vi "AIT 664 - Read End System XML.vi"(0 "Refnum in":refnum<k20>, 11 "error in (no error)":errorcluster) -> (4 "664 End System":T1, 15 "error out":errorcluster)   [LabVIEW 2013, in "AIT 664 Custom Device.lvlib"]
doc: "Read all of the nodes of the end system from xml configuration"
uses:
  AIT 664 Custom Device.lvlib
  Controls/664 - XML End System Description.ctl
  Controls/664 - XML Output VL.ctl
  Controls/664 - XML Tx Message Port.ctl
  Controls/664 - Sampling Type.ctl
  Controls/664 -Param.ctl
  Controls/664 - XML Input VL.ctl
  Controls/664 - XML Rx Message Port.ctl
  <vilib>/xml/Close Reference(NNMap).vi
  <vilib>/xml/Close Reference(Node).vi
  <resource>/objmgr/DOMUserDefRef.rc
  <vilib>/xml/NI_XML.lvlib
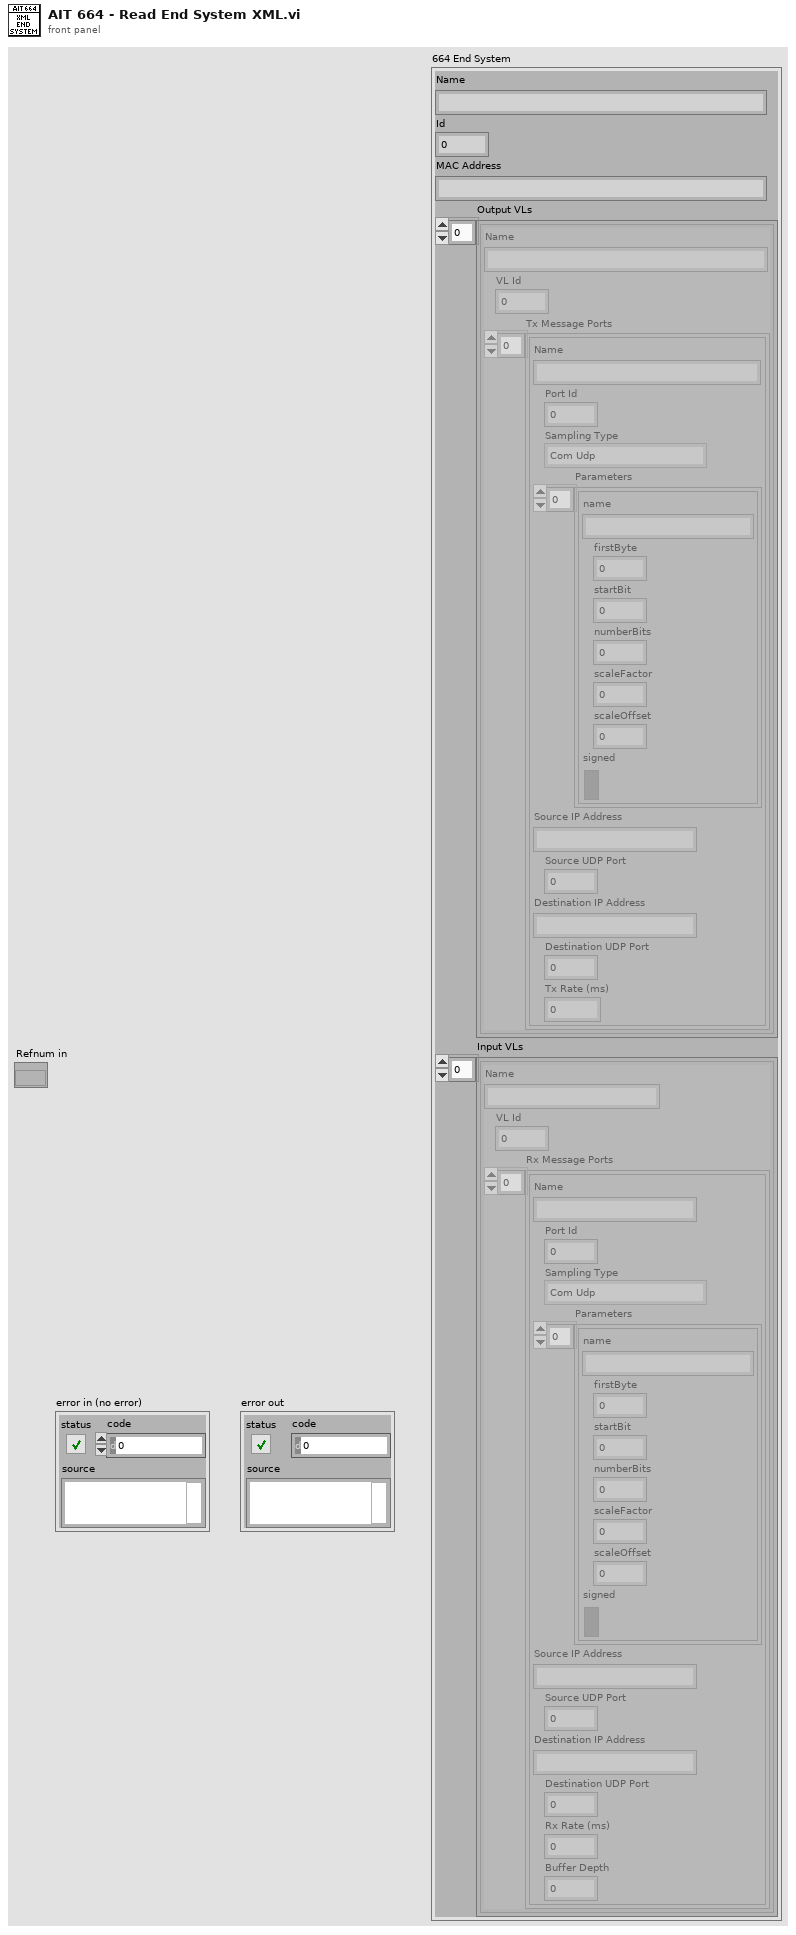
[diagram p1: front panel]
types:
  T1 = typedef "AIT 664 Custom Device.lvlib/664 - XML End System Description.ctl" = cluster{"Name":string, "Id":u32, "MAC Address":string, "Output VLs":T2[], "Input VLs":T6[]}
  T2 = typedef "AIT 664 Custom Device.lvlib/664 - XML Output VL.ctl" = cluster{"Name":string, "VL Id":u32, "Tx Message Ports":T3[]}
  T3 = typedef "AIT 664 Custom Device.lvlib/664 - XML Tx Message Port.ctl" = cluster{"Name":string, "Port Id":u32, "Sampling Type":T4, "Parameters":T5[], "Source IP Address":string, "Source UDP Port":u32, "Destination IP Address":string, "Destination UDP Port":u32, "Tx Rate (ms)":u32}
  T4 = typedef "AIT 664 Custom Device.lvlib/664 - Sampling Type.ctl" = enum16{"Com Udp", "Com Udp Queuing", "Sap Udp", "Sap Ip", "Sap Mac", "Unknown"}
  T5 = typedef "AIT 664 Custom Device.lvlib/664 -Param.ctl" = cluster{"name":string, "firstByte":i32, "startBit":i32, "numberBits":i32, "scaleFactor":dbl, "scaleOffset":dbl, "signed":bool}
  T6 = typedef "AIT 664 Custom Device.lvlib/664 - XML Input VL.ctl" = cluster{"Name":string, "VL Id":u32, "Rx Message Ports":T7[]}
  T7 = typedef "AIT 664 Custom Device.lvlib/664 - XML Rx Message Port.ctl" = cluster{"Name":string, "Port Id":u32, "Sampling Type":T4, "Parameters":T5[], "Source IP Address":string, "Source UDP Port":u32, "Destination IP Address":string, "Destination UDP Port":u32, "Rx Rate (ms)":u32, "Buffer Depth":u32}
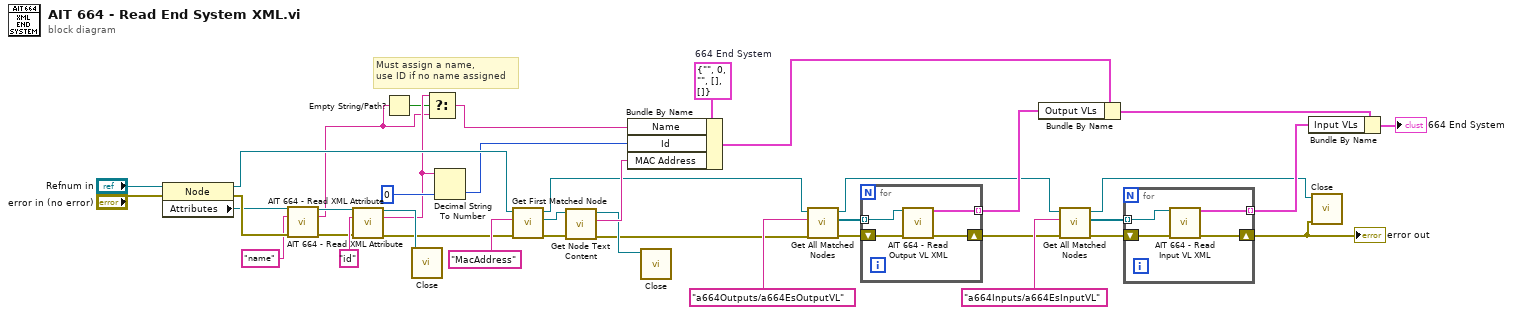
[diagram p0: block diagram]
diagram:
  w32 = T1 {"Name"="", "Id"=0, "MAC Address"="", "Output VLs"=[], "Input VLs"=[]}  # 664 End System
  # "Must assign a name,\nuse ID if no name assigned"
  n1 = property class="Node"(reference="Refnum in", error in="error in (no error)") -> (reference out=w40:refnum<k20>, error out=w27:errorcluster, "Attributes"=w24:refnum<k20>)
  n2 = call "AIT 664 - Read XML Attribute.vi"("Attributes In"=w24, "Attribute Name"="name", "error in (no error)"=w27) -> ("Attributes Out"=w29:refnum<k20>, "Attribute Text"=w1:string, "error out"=w28:errorcluster)  [unwired: 10 in]
  n3 = call "AIT 664 - Read XML Attribute.vi"("Attributes In"=w29, "Attribute Name"="id", "error in (no error)"=w28) -> ("Attributes Out"=w30:refnum<k20>, "Attribute Text"=w4:string, "error out"=w17:errorcluster)  [unwired: 10 in]
  n4 = Empty String/Path?(string/path=w1) -> (empty?=w2:bool)
  n5 = call-poly <vilib>:"Close.vi"("named node map"=w30) -> ()  [unwired: 8 in, 1 out]
  n6 = Select(t=w4, s=w2, f=w1) -> (s? t:f=w3:string)
  n7 = Decimal String To Number(string=w4, default (0L)=u32 0 ("default (0 I32)")) -> (number=w34:u32)  [unwired: 1 in, 1 out]
  n8 = call <vilib>:"Get First Matched Node.vi"("error in (no error)"=w17, "XPath expression"="MacAddress", "node in"=w40) -> ("error out"=w39:errorcluster, "node result"=w37:refnum<k20>, "node out"=w12:refnum<k20>)  [unwired: 6 in]
  n9 = call <vilib>:"Get Node Text Content.vi"("error in (no error)"=w39, "node in"=w37) -> ("error out"=w16:errorcluster, "node text"=w38:string, "node out"=w23:refnum<k20>)  [unwired: 7 in]
  n10 = Bundle By Name(cluster=w32, "Name"=w3, "Id"=w34, "MAC Address"=w38) -> (w19:T1)
  n11 = call-poly <vilib>:"Close.vi"("node"=w23) -> ()  [unwired: 8 in, 1 out]
  n12 = call <vilib>:"Get All Matched Nodes.vi"("error in (no error)"=w16, "XPath expression"="a664Outputs/a664EsOutputVL", "node in"=w12) -> ("error out"=w20:errorcluster, "node result array"=w21:refnum<k20>[], "node out"=w11:refnum<k20>)  [unwired: 6 in]
  n13 = for {
    tunnel: w21 -> [w42] mode=indexing
    tunnel: [w41] -> w18 mode=indexing
    shift-right: [w43] -> w10
    shift-left: w20 -> [w44]
    n14 = call "AIT 664 - Read Output VL XML.vi"("Node Reg"=w42, "error in (no error)"=w44) -> ("Output VL"=w41:T2, "error out"=w43:errorcluster)  [unwired: 12 in]
  }
  n15 = Bundle By Name(cluster=w19, "Output VLs"=w18) -> (w8:T1)
  n16 = call <vilib>:"Get All Matched Nodes.vi"("error in (no error)"=w10, "XPath expression"="a664Inputs/a664EsInputVL", "node in"=w11) -> ("error out"=w13:errorcluster, "node result array"=w14:refnum<k20>[], "node out"=w5:refnum<k20>)  [unwired: 6 in]
  n17 = for {
    tunnel: w14 -> [w48] mode=indexing
    tunnel: [w46] -> w9 mode=indexing
    shift-right: [w45] -> w6
    shift-left: w13 -> [w47]
    n18 = call "AIT 664 - Read Input VL XML.vi"("Refnum in"=w48, "error in (no error)"=w47) -> ("Input VL"=w46:T6, "error out"=w45:errorcluster)  [unwired: 12 in]
  }
  "error out" <- w6
  n19 = Bundle By Name(cluster=w8, "Input VLs"=w9) -> (→"664 End System":T1)
  n20 = call-poly <vilib>:"Close.vi"("error in (no error)"=w6, "node"=w5) -> ()  [unwired: 7 in, 1 out]
